vi "Prueba_mensajes_WRD.vi"() -> ()   [LabVIEW 2015]
panel:
  out "date/time string":string
  out "Report_AURA":string
  out "Report":string
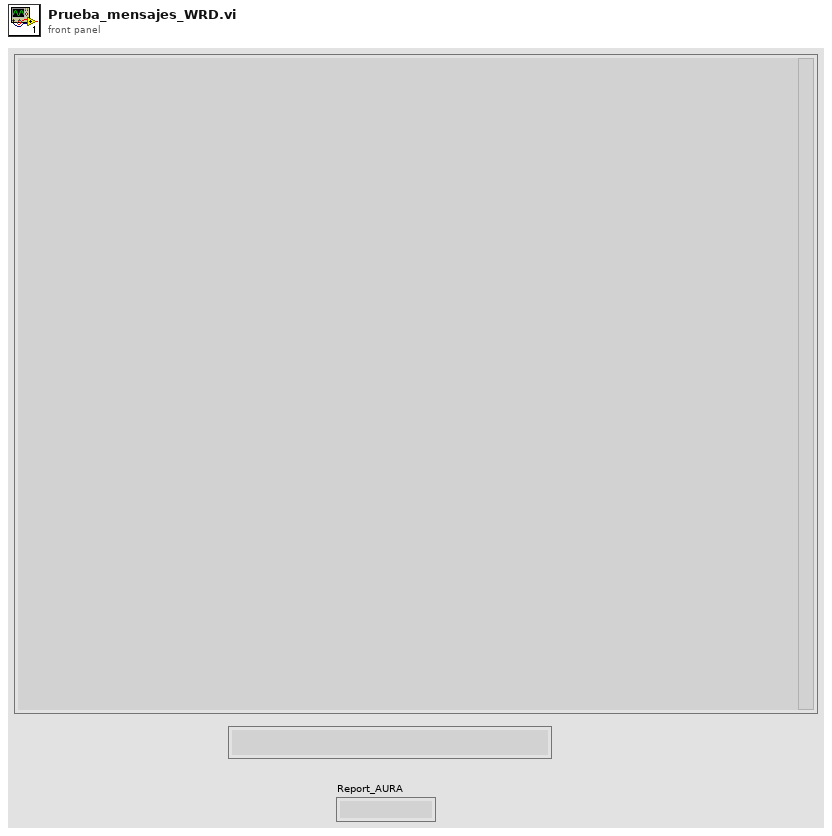
[diagram p1: front panel]
types:
  T1 = cluster{"error out":errorcluster, dbl[], "TAGs":string[], "Direccion 0?":bool}
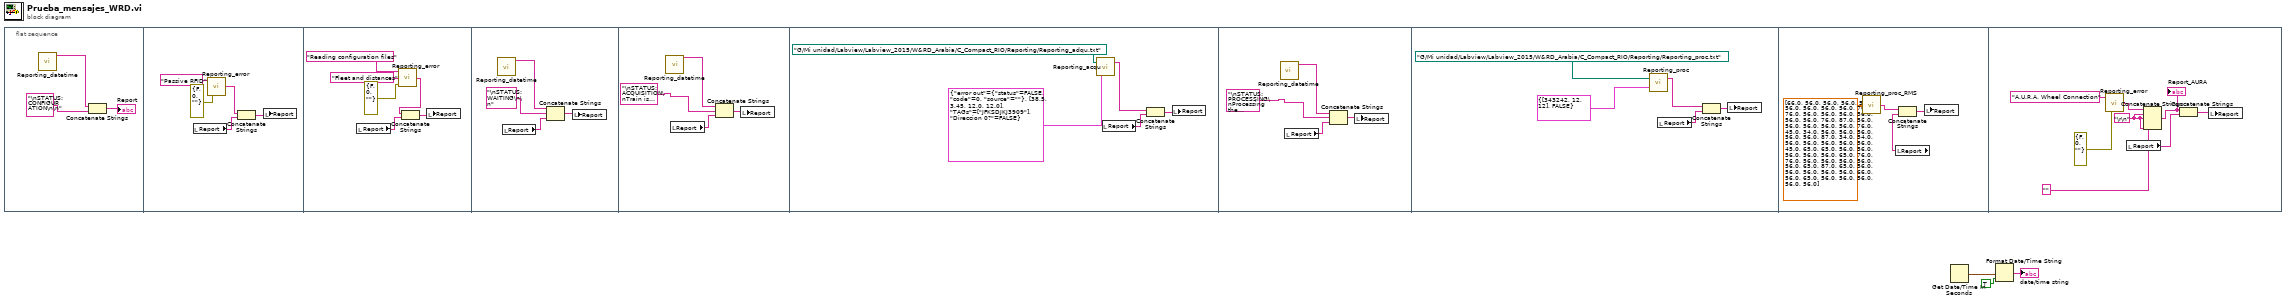
[diagram p0: block diagram]
diagram:
  n1 = flat-sequence {
    frame #0 {
      n2 = call "Reporting_datetime.vi"() -> ("String"=w6:string)  [unwired: 11 in]
      n3 = Concatenate Strings(w6, "\nSTATUS: CONFIGURATION\n\n") -> (→"Report":string)
    }
    frame #1 {
      n4 = local read "Report"() -> (w11:string)
      n5 = call "Reporting_error.vi"("error out 2"=errorcluster {"status"=FALSE, "code"=0, "source"=""}, "Concept"="Passive RFID") -> ("Reporting"=w8:string)  [unwired: 1 in]
      n6 = Concatenate Strings(w8, w11) -> (w10:string)
      n7 = local write "Report"(w10) -> ()
    }
    frame #2 {
      n8 = local read "Report"() -> (w16:string)
      n9 = call "Reporting_error.vi"("error out 2"=errorcluster {"status"=FALSE, "code"=0, "source"=""}, "Concept explanation"="Fleet and distances", "Concept"="Reading configuration files") -> ("Reporting"=w13:string)
      n10 = Concatenate Strings(w13, w16) -> (w17:string)
      n11 = local write "Report"(w17) -> ()
    }
    frame #3 {
      n12 = call "Reporting_datetime.vi"() -> ("String"=w18:string)  [unwired: 11 in]
      n13 = local read "Report"() -> (w20:string)
      n14 = Concatenate Strings(w18, "\nSTATUS: WAITING\n\n", w20) -> (w21:string)
      n15 = local write "Report"(w21) -> ()
    }
    frame #4 {
      n16 = call "Reporting_datetime.vi"() -> ("String"=w25:string)  [unwired: 11 in]
      n17 = local read "Report"() -> (w24:string)
      n18 = Concatenate Strings(w25, "\nSTATUS: ACQUISITION\nTrain is passing\n\n", w24) -> (w23:string)
      n19 = local write "Report"(w23) -> ()
    }
    frame #5 {
      n20 = call "Reporting_acqu.vi"("output cluster"=T1 {"error out"={"status"=FALSE, "code"=0, "source"=""}, [38.5, 3.45, 12.0, 12.0], "TAGs"=["JFKSDJKJ3909"], "Direccion 0?"=FALSE}, "address repoting"=path "G:/Mi unidad/Labview/Labview_2015/W&RD_Arabia/C_Compact_RIO/Reporting/Reporting_adqu.txt" ("file (use dialog)")) -> ("Reporting"=w26:string)  [unwired: 1 in]
      n21 = local read "Report"() -> (w29:string)
      n22 = Concatenate Strings(w26, w29) -> (w30:string)
      n23 = local write "Report"(w30) -> ()
    }
    frame #6 {
      n24 = call "Reporting_datetime.vi"() -> ("String"=w34:string)  [unwired: 11 in]
      n25 = local read "Report"() -> (w33:string)
      n26 = Concatenate Strings(w34, "\nSTATUS: PROCESSING\nProcessing the measurement\n\n", w33) -> (w32:string)
      n27 = local write "Report"(w32) -> ()
    }
    frame #7 {
      n28 = call "Reporting_proc.vi"("output cluster 2"=cluster{i64[], bool} {[343242, 12, 12], FALSE}, "address repoting"=path "G:/Mi unidad/Labview/Labview_2015/W&RD_Arabia/C_Compact_RIO/Reporting/Reporting_proc.txt" ("file (use dialog)")) -> ("Reporting"=w35:string)  [unwired: 1 in]
      n29 = local read "Report"() -> (w36:string)
      n30 = Concatenate Strings(w35, w36) -> (w37:string)
      n31 = local write "Report"(w37) -> ()
    }
    frame #8 {
      n32 = call "Reporting_proc_RMS.vi"("Max RMS Ruedas"=dbl[][] [[66.0, 56.0, 56.0, 56.0, 56.0, 56.0, 56.0, 56.0], [56.0, 76.0, 76.0, 56.0, 56.0, 56.0, 56.0, 56.0], [56.0, 76.0, 87.0, 56.0, 56.0, 56.0, 56.0, 56.0], [76.0, 45.0, 34.0, 56.0, 56.0, 56.0, 56.0, 56.0], [87.0, 34.0, 54.0, 56.0, 56.0, 56.0, 56.0, 56.0], [45.0, 65.0, 65.0, 56.0, 56.0, 56.0, 56.0, 56.0], [65.0, 76.0, 76.0, 56.0, 56.0, 56.0, 56.0, 56.0], [65.0, 87.0, 65.0, 56.0, 56.0, 56.0, 56.0, 56.0], [66.0, 56.0, 65.0, 56.0, 56.0, 56.0, 56.0, 56.0]]) -> ("String"=w41:string)
      n33 = local read "Report"() -> (w43:string)
      n34 = Concatenate Strings(w41, w43) -> (w42:string)
      n35 = local write "Report"(w42) -> ()
    }
    frame #9 {
      w50 = "\r\n"
      n36 = call "Reporting_error.vi"("error out 2"=errorcluster {"status"=FALSE, "code"=0, "source"=""}, "Concept"="A.U.R.A. Wheel Connection") -> ("Reporting"=w51:string)  [unwired: 1 in]
      n37 = local read "Report"() -> (w47:string)
      n38 = Concatenate Strings(w51, w50, w50, "" ("string"), w50) -> (w49:string)
      "Report_AURA" <- w49
      n39 = Concatenate Strings(w49, w47) -> (w48:string)
      n40 = local write "Report"(w48) -> ()
    }
  }
  n41 = Get Date/Time In Seconds() -> (seconds since 1Jan1904=w2:timestamp)
  n42 = Format Date/Time String(seconds (now)=w2, UTC format=TRUE) -> (date/time string=→"date/time string":string)  [unwired: 1 in]
